vi "Convert Bool Array to Cluster BLOB.vi"(7 "Total Bytes":i32, 8 "error in (no error)":errorcluster, 9 "Cluster Bool Array out":bool[](array[boolean]), 10 "Byte array":u8[](array[numeric])) -> (0 "error out":errorcluster, 2 "Cluster BLOB":u8[](array[numeric]))   [LabVIEW 2020, in "FPGA Register IO.lvlib"]
uses:
  FPGA Register IO.lvlib
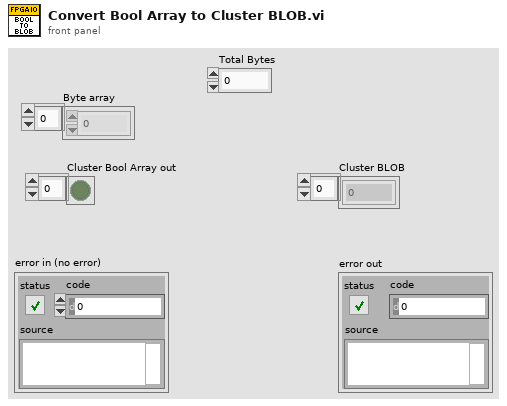
[diagram p1: front panel]
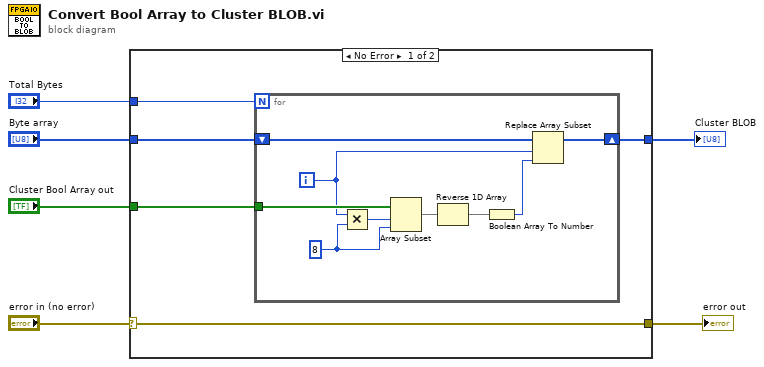
[diagram p0: block diagram]
diagram:
  n1 = case shown="No Error" "error in (no error)" {
    selector: "error in (no error)" -> [w11 w21]
    tunnel: [w11 w21] -> w5
    tunnel: "Cluster Bool Array out" -> [w9 _]
    tunnel: [w10 _] -> w3
    tunnel: "Total Bytes" -> [w8 _]
    tunnel: "Byte array" -> [w7 _]
    frame No Error {
      n2 = for {
        N: w8 -> [_]
        tunnel: w9 -> [w20]
        shift-right: [w18] -> w10
        shift-left: w7 -> [w19]
        i -> [w15]
        w14 = 8 ("length")
        n3 = Multiply(x=w15, y=w14) -> (x*y=w17:i32)
        n4 = Array Subset(array=w20, index=w17, length=w14) -> (w13:bool[])
        n5 = Reverse 1D Array(array=w13) -> (reversed array=w12:bool[])
        n6 = Boolean Array To Number(Boolean array=w12) -> (number=w16:u8)
        n7 = Replace Array Subset(array=w19, new element=w16, index=w15) -> (w18:u8[])
      }
    }
    frame Error {
    }
  }
  "error out" <- w5
  "Cluster BLOB" <- w3
